vi "Fit phase one.vi"(9 "Initial parameters":dbl[](array[numeric])=[188.484, 0.01, 2.4] format="%#_6p", 10 "Z":cdb[](array[numeric]), 11 "X":dbl[](array[numeric])) -> ()   [LabVIEW 2016]
uses:
  <vilib>/gmath/NumericalOptimization/Nonlinear Curve Fit LM bound.vi
  <vilib>/gmath/NI_Gmath.lvlib
panel:
  out "XY Graph 3":cluster{"X":dbl[], dbl[]}(graph)
  out "XY Graph 2":cluster{"X":dbl[], dbl[]}(graph)
  out "XY Graph":cluster{"X":dbl[], dbl[]}(graph)
  in  "Bounds":T1={"parameter minimum"=[188.0, 0.0001, 0.0], "parameter maximum"=[189.0, 0.01, 3.15]} {"parameter minimum" format="%#_6p"}
  out "Weight":dbl[](graph)
  out "best fit parameters":dbl[](array[numeric]) format="%#_6p"
  out "number of function calls":i32
  in  "termination":cluster{"max iteration":i32, "tolerance":dbl}={"max iteration"=200, "tolerance"=1e-08}
  out "Fit":cluster{"X":dbl[], "best nonlinear fit":dbl[]}[](graph)
  # "F0\nG\nA\nP\nX\nY"
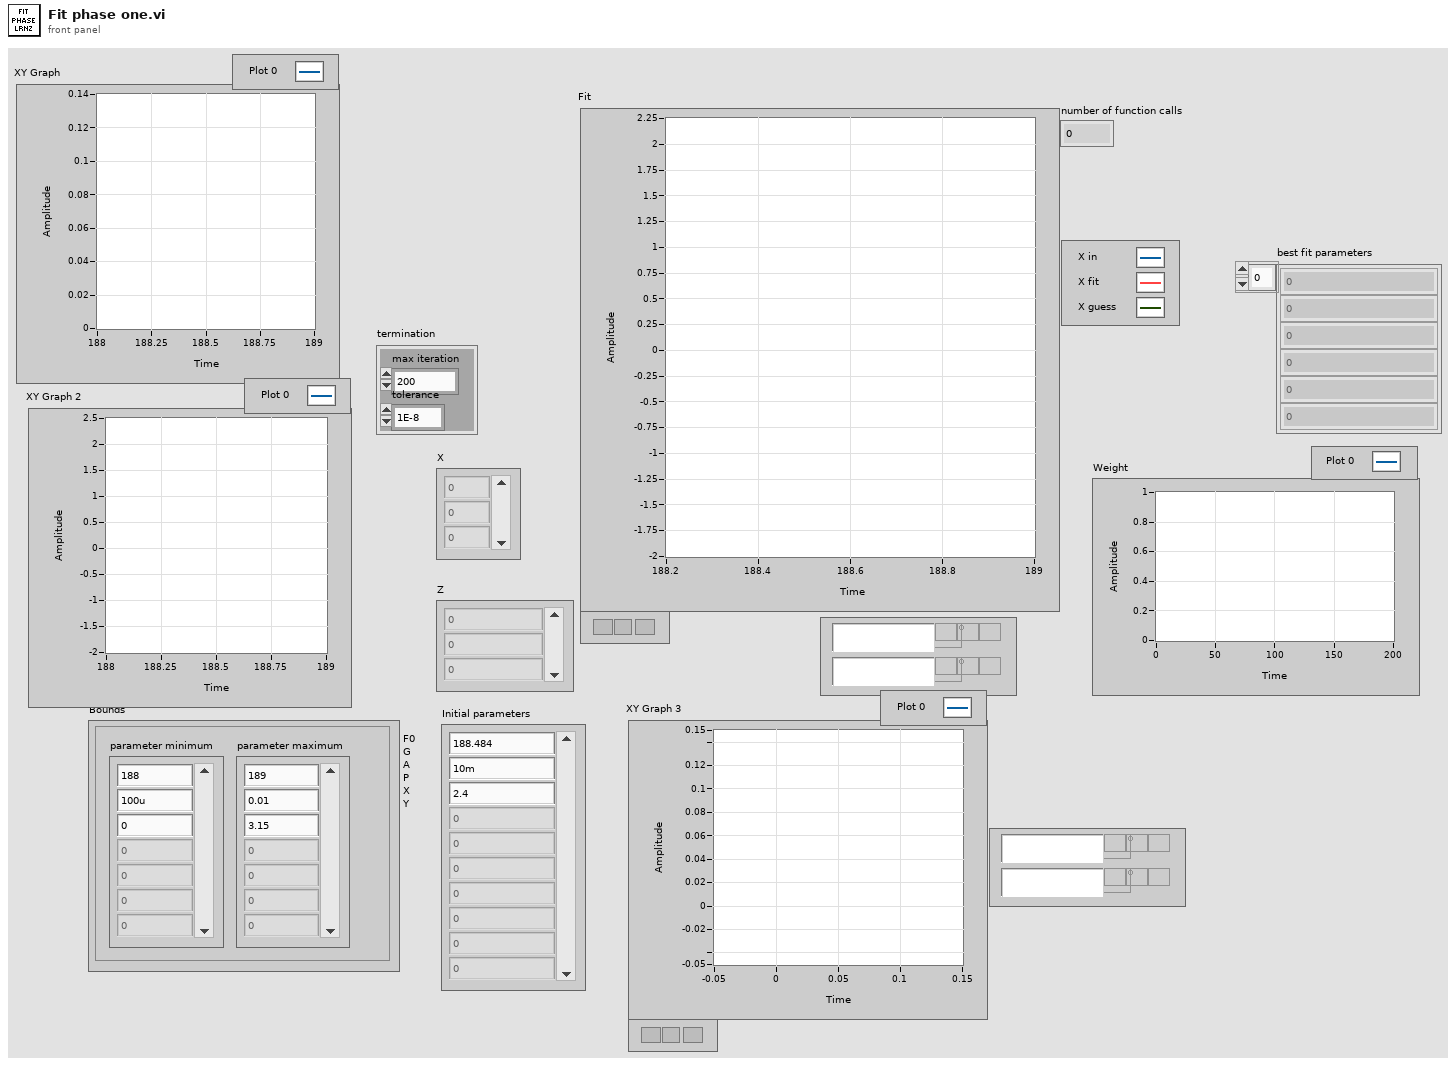
[diagram p1: front panel]
types:
  T1 = cluster{"parameter minimum":dbl[], "parameter maximum":dbl[]}
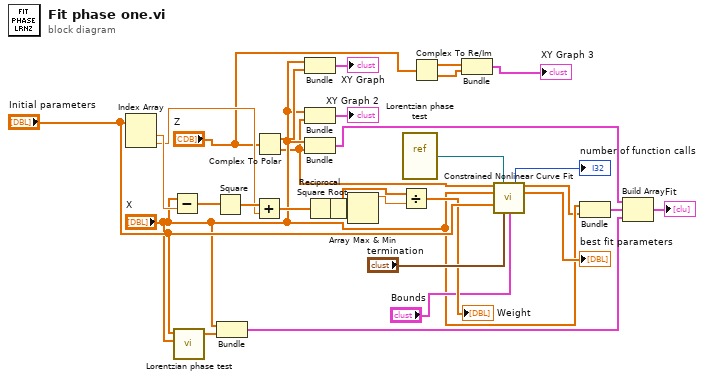
[diagram p0: block diagram]
diagram:
  n1 = Index Array(array="Initial parameters") -> (element #1=w20:dbl, element #2=w17:dbl)  [unwired: 2 in]
  n2 = Subtract(x="X", y=w20) -> (x-y=w19:dbl[])
  n3 = call "Lorentzian phase test.vi"("X"="X", "a"="Initial parameters") -> ("f(X,a)"=w22:dbl[])  [unwired: 2 in, 2 out]
  n4 = Square(x=w19) -> (x^2=w18:dbl[])
  n5 = Bundle("X"="X", "f(X,a)"=w22) -> (w25:cluster{"X":dbl[], "f(X,a)":dbl[]})  [unwired: 1 in]
  n6 = Add(x=w18, y=w17) -> (x+y=w16:dbl[])
  n7 = Complex To Polar(r * e^(i*theta)="Z") -> (r=w11:dbl[], theta=w7:dbl[])
  n8 = Bundle("X"="X", w11) -> (→"XY Graph":cluster{"X":dbl[], dbl[]})  [unwired: 1 in]
  n9 = Bundle("X"="X", w7) -> (→"XY Graph 2":cluster{"X":dbl[], dbl[]})  [unwired: 1 in]
  n10 = Bundle("X"="X", w7) -> (w24:cluster{"X":dbl[], dbl[]})  [unwired: 1 in]
  n11 = Reciprocal(x=w16) -> (1/x=w14:dbl[])
  n12 = Square Root(x=w14) -> (sqrt(x)=w1:dbl[])
  n13 = Array Max & Min(array=w1) -> (max value=w13:dbl)  [unwired: 3 out]
  n14 = Divide(x=w1, y=w13) -> (x/y=→"Weight":dbl[])
  n15 = vi-ref "Lorentzian phase test.vi"() -> (w30:refnum<vi>)
  n16 = Complex To Re/Im(x + iy="Z") -> (x=w4:dbl[], y=w3:dbl[])
  n17 = Bundle(w4, w3) -> (→"XY Graph 3":cluster{dbl[], dbl[]})  [unwired: 1 in]
  n18 = call-poly <vilib>:"Constrained Nonlinear Curve Fit.vi"("Y"=w7, "f(x,a)"=w30, "X"="X", "initial parameters"="Initial parameters", "termination"="termination", "parameter bounds"="Bounds") -> ("number of function calls"=→"number of function calls":i32, "best nonlinear fit"=w6:dbl[], "best fit parameters"=→"best fit parameters":dbl[])  [unwired: 4 in, 3 out]
  n19 = Bundle("X"="X", "best nonlinear fit"=w6) -> (w23:cluster{"X":dbl[], "best nonlinear fit":dbl[]})  [unwired: 1 in]
  n20 = Build Array(w24, w23, w25) -> (→"Fit":cluster{"X":dbl[], "f(X,a)":dbl[]}[])
